vi "Go-NoGo.vi"(8 "error in (no error)":errorcluster, 9 "Go-NoGo Data":variant, 10 "Go?":bool, 11 "Father of all uServices in":refnum<class "Father of all uServices.lvclass">) -> (0 "error out":errorcluster, 3 "Father of all uServices out":refnum<class "Father of all uServices.lvclass">)   [LabVIEW 2026, in "TALOS.lvlib" / "Father of all uServices.lvlib" / "Father of all uServices.lvclass"]
doc: "This VI reports the status of the initial check perform during the Ready to launch? routine."
uses:
  Father of all uServices.lvclass
  C:/LabVIEW Code/TALOS/talos/Ancestor/Ancestor/Ancestor.lvclass
  C:/LabVIEW Code/TALOS/builds/Actor Framework PPL/Actor Framework.lvlibp/1abvi3w/vi.lib/ActorFramework/Actor/Actor.lvclass
  Support VIs/Go-NoGo.ctl
  Ancestor/Ancestor/Ancestor.lvclass/Ancestor.ctl
  Guardian/Guardian Messages/Message to uService Msg/Message to uService Msg.lvclass/Message to uService Msg.ctl
  Ancestor/Ancestor/Read ID.vi
  Guardian/Guardian Messages/Message to uService Msg/Send Message to uService.vi
  Support VIs/Substitute Error.vi
  Support VIs/Generate Error.vi
  FGV/Error Memory/Get Error Description.vi
  Support VIs/Get PC name.vi
  Support VIs/Get Class Name.vi
  <vilib>/Utility/error.llb/Clear Errors.vi
  FGV/Error Memory/Error Memory Core.vi
  <vilib>/AdvancedString/Delimited String to 1D String Array.vi
  <vilib>/AdvancedString/Delimited String to 1D String Array (string).vi
  Support VIs/Circus Root Path.vi
  FGV/Error Memory/Error Crt Lvl checker.vi
  FGV/Error Memory/Error Memory Core.vi/40c8088d-b597-4017-91af-faa98e00292e.vi
  FGV/Error Memory/Error Memory Core.vi/d4a3ab98-063c-4e44-b43d-fbdcfe6c2be2.vi
  Support VIs/Global Constants.vi
  builds/Actor Framework PPL/Actor Framework.lvlibp/1abvi3w/vi.lib/ActorFramework/Actor/Read Caller Enqueuer.vi
  builds/Actor Framework PPL/Actor Framework.lvlibp/1abvi3w/vi.lib/ActorFramework/Message Enqueuer/Enqueue.vi
  Support VIs/Global Memory.vi
  <vilib>/Utility/LVClass/Get LV Class Name.vi
  Support VIs/Is in Packed Library.vi
  Support VIs/TALOS Root path.vi
  Support VIs/Read CSV worksheet.vi
  <vilib>/Utility/error.llb/General Error Handler.vi
  Support VIs/Error Log.vi
  Guardian/Guardian Messages/Message to uService Msg/Message to uService Msg.lvclass
  Ancestor/Ancestor/Ancestor.lvclass
  <vilib>/Comparison/Equal/Equal Functor/Equal Functor.lvclass
  TALOS.lvlib
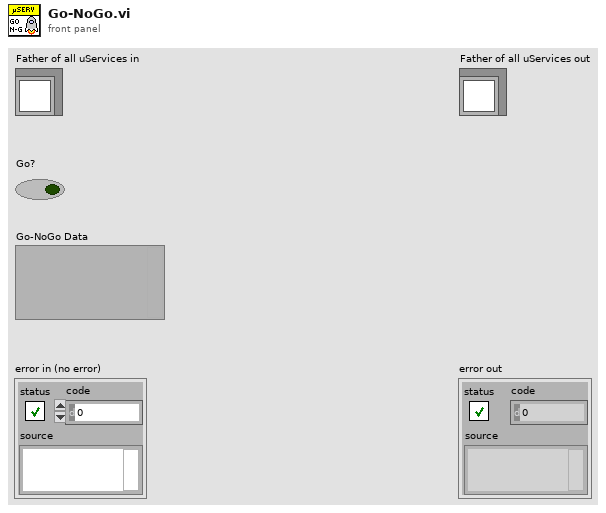
[diagram p1: front panel]
types:
  T1 = typedef "TALOS.lvlib/Go-NoGo.ctl" = cluster{"ID":string, "Status":bool, "Data":string[], "GUID":string}
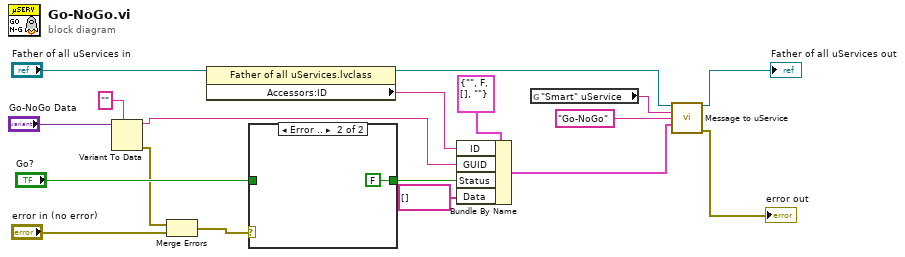
[diagram p0: block diagram]
diagram:
  n1 = Variant To Data(type="", Variant="Go-NoGo Data") -> (data=w3:string, error out=w4:errorcluster)  [unwired: 1 in]
  n2 = Merge Errors(w4, "error in (no error)") -> (w5:errorcluster)
  n3 = property class="Father of all uServices.lvclass"(reference="Father of all uServices in") -> (reference out=w14:refnum<class "Father of all uServices.lvclass">, "Accessors:ID"=w8:string)  [unwired: 1 in, 1 out]
  n4 = case shown="Error .." w5 {
    tunnel: "Go?" -> [w19 _]
    tunnel: [w19 FALSE ("Go?")] -> w11
    frame No Error {
    }
    frame Error {
    }
  }
  n5 = Bundle By Name(cluster=T1 {"ID"="", "Status"=FALSE, "Data"=[], "GUID"=""} ("Go-NoGo"), "ID"=w8, "GUID"=w3, "Status"=w11, "Data"=string[] []) -> (w10:T1)
  n6 = global read "Global Constants.vi" "\"Smart\" uService"() -> (w2:string)
  n7 = call "Message to uService.vi"("Father of all uServices in"=w14, "uService ID"=w2, "Message"="Go-NoGo", "Data"=w10) -> ("Father of all uServices out"=→"Father of all uServices out":refnum<class "Father of all uServices.lvclass">, "error out"=→"error out":errorcluster)  [unwired: 10 in]
